vi "kinesis_test.vi"() -> ()   [LabVIEW 2015]
uses:
  thorlabs_drivers/Thorlabs.MotionControl.Benchtop.Piezo.dll
panel:
  in  "newpos":i16
  in  "stop":bool
  out "return type 7":i16
  out "return type 6":i16
  out "return type 5":i8
  out "return type 4":i16
  out "return type 3":i16
  out "return type 2":i16
  out "error out":errorcluster
  out "return type":i16
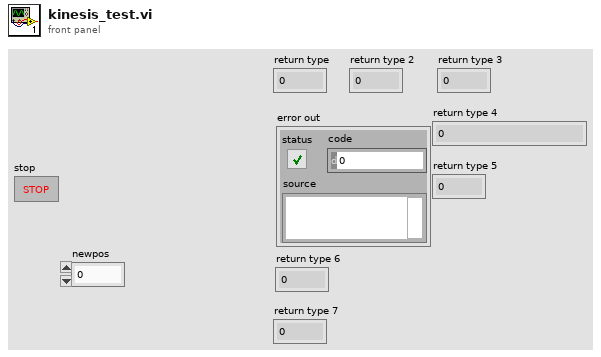
[diagram p1: front panel]
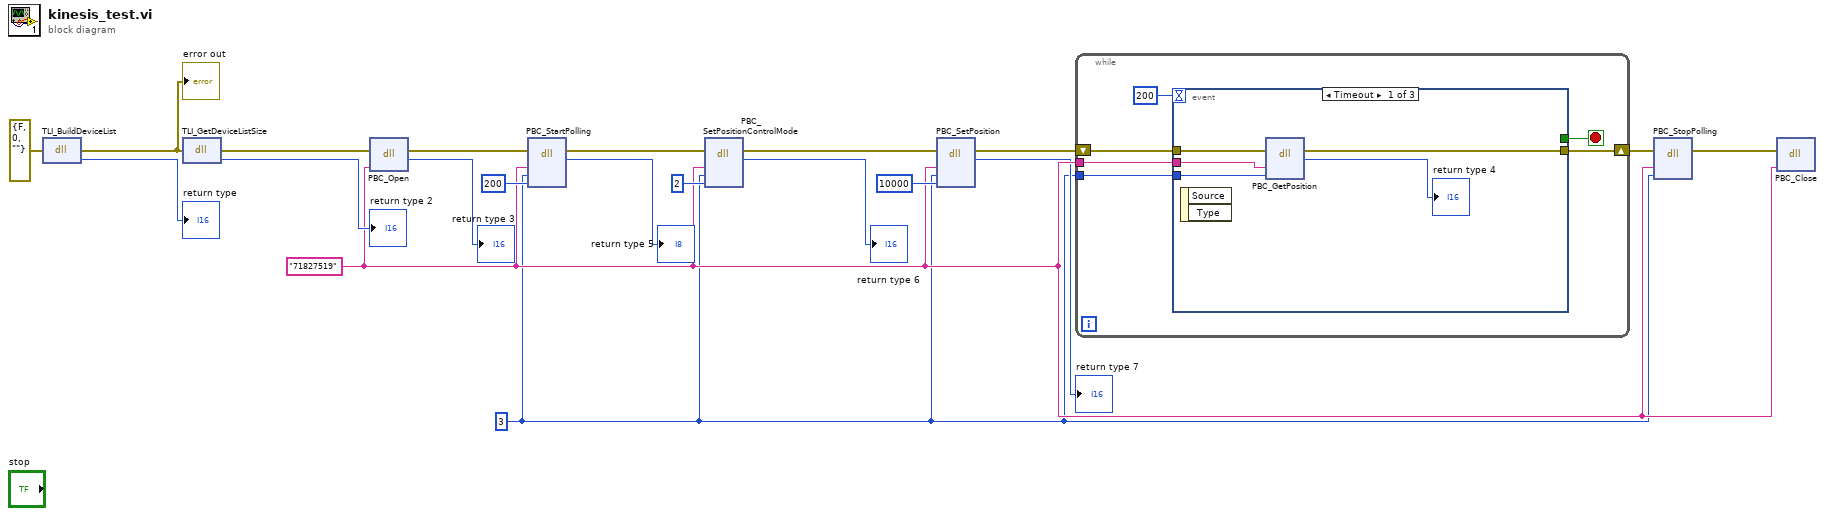
[diagram p0: block diagram]
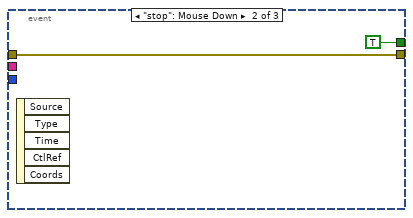
[diagram p2: hidden frame]
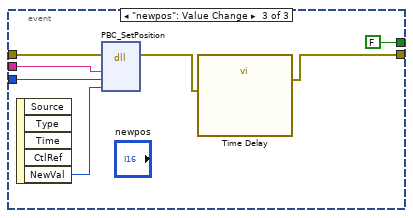
[diagram p3: hidden frame]
diagram:
  w1 = i16 3 ("channel")
  w5 = "71827519" ("serialNo")
  n1 = dll-call lib="C:/Users/MX-Microscope/Documents/LabVIEW Data/pcfs_lvoop_2017-master_170904/Stage Class/Thorlabs Kinesis/thorlabs_drivers/Thorlabs.MotionControl.Benchtop.Piezo.dll" fn="TLI_BuildDeviceList"(error in=errorcluster {"status"=FALSE, "code"=0, "source"=""} ("error in (no error)")) -> (error out=w17:errorcluster, "return type"=→"return type":i16)  [unwired: 2 in, 1 out]
  "error out" <- w17
  n2 = dll-call lib="C:/Users/MX-Microscope/Documents/LabVIEW Data/pcfs_lvoop_2017-master_170904/Stage Class/Thorlabs Kinesis/thorlabs_drivers/Thorlabs.MotionControl.Benchtop.Piezo.dll" fn="TLI_GetDeviceListSize"(error in=w17) -> (error out=w16:errorcluster, "return type"=→"return type 2":i16)  [unwired: 2 in, 1 out]
  n3 = dll-call lib="C:/Users/MX-Microscope/Documents/LabVIEW Data/pcfs_lvoop_2017-master_170904/Stage Class/Thorlabs Kinesis/thorlabs_drivers/Thorlabs.MotionControl.Benchtop.Piezo.dll" fn="PBC_Open"(error in=w16, "serial"=w5) -> (error out=w14:errorcluster, "return type"=→"return type 3":i16)  [unwired: 3 in, 1 out]
  n4 = dll-call lib="C:/Users/MX-Microscope/Documents/LabVIEW Data/pcfs_lvoop_2017-master_170904/Stage Class/Thorlabs Kinesis/thorlabs_drivers/Thorlabs.MotionControl.Benchtop.Piezo.dll" fn="PBC_StartPolling"(error in=w14, "serial"=w5, "channel"=w1, "millisecs"=200) -> (error out=w11:errorcluster, "return type"=→"return type 5":i8)  [unwired: 5 in, 1 out]
  n5 = dll-call lib="C:/Users/MX-Microscope/Documents/LabVIEW Data/pcfs_lvoop_2017-master_170904/Stage Class/Thorlabs Kinesis/thorlabs_drivers/Thorlabs.MotionControl.Benchtop.Piezo.dll" fn="PBC_SetPositionControlMode" label="PBC_SetPositionMode"(error in=w11, "serial"=w5, "channel"=w1, "PositionControlMode"=i16 2) -> (error out=w9:errorcluster, "return type"=→"return type 6":i16)  [unwired: 5 in, 1 out]
  n6 = dll-call lib="C:/Users/MX-Microscope/Documents/LabVIEW Data/pcfs_lvoop_2017-master_170904/Stage Class/Thorlabs Kinesis/thorlabs_drivers/Thorlabs.MotionControl.Benchtop.Piezo.dll" fn="PBC_SetPosition"(error in=w9, "serial"=w5, "channel"=w1, "volts"=i16 10000 ("position")) -> (error out=w7:errorcluster, "return type"=→"return type 7":i16)  [unwired: 5 in, 1 out]
  n7 = while {
    tunnel: w5 -> [w24]
    shift-right: [w25] -> w6
    shift-left: w7 -> [w26]
    tunnel: w1 -> [w21]
    stop <- w22 stop-if-true
    n8 = event shown="[0] Timeout" {
      selector: _ -> [_ _ _]
      dyn-events: _ -> [_ _ _]
      timeout: 200 -> [_ _ _]
      tunnel: w26 -> [w31 w32 w39]
      tunnel: [w30 w32 w36] -> w25
      tunnel: w24 -> [w29 _ w40]
      tunnel: [_ TRUE FALSE] -> w22
      tunnel: w21 -> [w27 _ w35]
      event Timeout {
        n9 = event-data() -> ()  [unwired: 1 in, 2 out]
        n10 = dll-call lib="C:/Users/MX-Microscope/Documents/LabVIEW Data/pcfs_lvoop_2017-master_170904/Stage Class/Thorlabs Kinesis/thorlabs_drivers/Thorlabs.MotionControl.Benchtop.Piezo.dll" fn="PBC_GetPosition" label="PBC_GetOutputVoltage"(error in=w31, "serial"=w29, "channel"=w27) -> (error out=w30:errorcluster, "return type"=→"return type 4":i16)  [unwired: 4 in, 1 out]
      }
      event "stop": Mouse Down {
        n11 = event-data() -> ()  [unwired: 1 in, 5 out]
      }
      event "newpos": Value Change {
        n12 = event-data() -> ("NewVal"=w34:i16)  [unwired: 1 in, 4 out]
        n13 = dll-call lib="C:/Users/MX-Microscope/Documents/LabVIEW Data/pcfs_lvoop_2017-master_170904/Stage Class/Thorlabs Kinesis/thorlabs_drivers/Thorlabs.MotionControl.Benchtop.Piezo.dll" fn="PBC_SetPosition"(error in=w39, "serial"=w40, "channel"=w35, "volts"=w34) -> (error out=w37:errorcluster)  [unwired: 6 in, 1 out]
        n14 = call "Time Delay"("error in (no error)"=w37) -> ("error out"=w36:errorcluster)  [unwired: 10 in]
      }
    }
  }
  n15 = dll-call lib="C:/Users/MX-Microscope/Documents/LabVIEW Data/pcfs_lvoop_2017-master_170904/Stage Class/Thorlabs Kinesis/thorlabs_drivers/Thorlabs.MotionControl.Benchtop.Piezo.dll" fn="PBC_StopPolling"(error in=w6, "serial"=w5, "channel"=w1) -> (error out=w12:errorcluster)  [unwired: 5 in, 1 out]
  n16 = dll-call lib="C:/Users/MX-Microscope/Documents/LabVIEW Data/pcfs_lvoop_2017-master_170904/Stage Class/Thorlabs Kinesis/thorlabs_drivers/Thorlabs.MotionControl.Benchtop.Piezo.dll" fn="PBC_Close"(error in=w12, "serial"=w5) -> ()  [unwired: 4 in, 2 out]
